vi "VsEP-Compute Final Average.vi"(0 "#Avgs":i32, 1 "Remove DC Offset":bool=TRUE, 5 "Running Sum 1":dbl[](array[numeric]), 9 "Running Sum 2":dbl[](array[numeric]), 11 "AltPol":bool) -> (6 "Neural":dbl[](array[numeric]), 10 "Microphonic":dbl[](array[numeric]))   [LabVIEW 2020]
uses:
  <vilib>/Analysis/baseanly.llb/Mean (DBL).vi
  <vilib>/Analysis/NI_AALBase.lvlib
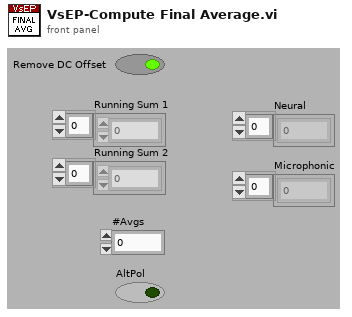
[diagram p1: front panel]
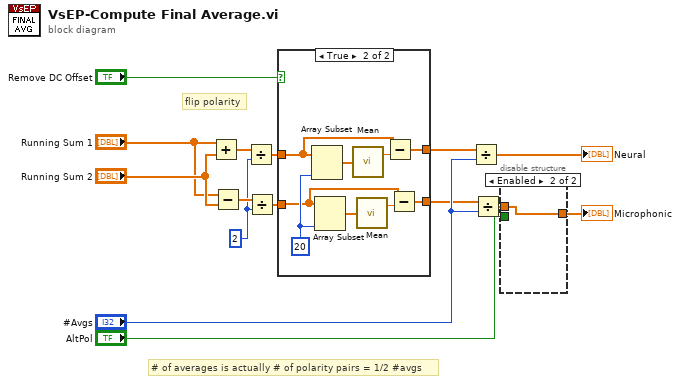
[diagram p0: block diagram]
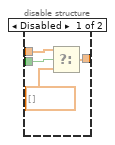
[diagram p3: hidden frame]
diagram:
  w1 = 2
  # "flip polarity"
  # "# of averages is actually # of polarity pairs = 1/2 #avgs"
  n1 = Add(x="Running Sum 1", y="Running Sum 2") -> (x+y=w5:dbl[])
  n2 = Subtract(x="Running Sum 1", y="Running Sum 2") -> (x-y=w4:dbl[])
  n3 = Divide(x=w5, y=w1) -> (x/y=w3:dbl[])
  n4 = Divide(x=w4, y=w1) -> (x/y=w2:dbl[])
  n5 = case shown="True" "Remove DC Offset" {
    tunnel: [w17 w21] -> w8
    tunnel: w3 -> [w17 w22]
    tunnel: [w16 w18] -> w9
    tunnel: w2 -> [w16 w20]
    frame False {
    }
    frame True {
      w26 = 20
      n6 = Array Subset(array=w22, length=w26) -> (w24:dbl[])  [unwired: 1 in]
      n7 = Array Subset(array=w20, length=w26) -> (w25:dbl[])  [unwired: 1 in]
      n8 = call-poly <vilib>:"Mean.vi"("X"=w24) -> ("mean"=w23:dbl)  [unwired: 1 out]
      n9 = call-poly <vilib>:"Mean.vi"("X"=w25) -> ("mean"=w19:dbl)  [unwired: 1 out]
      n10 = Subtract(x=w22, y=w23) -> (x-y=w21:dbl[])
      n11 = Subtract(x=w20, y=w19) -> (x-y=w18:dbl[])
    }
  }
  n12 = Divide(x=w8, y="#Avgs") -> (x/y=→"Neural":dbl[])
  n13 = Divide(x=w9, y="#Avgs") -> (x/y=w11:dbl[])
  n14 = disable-structure shown="Enabled" {
    disable-tunnel: "AltPol" -> [w30 _]
    disable-tunnel: [w28 w31] -> w12
    disable-tunnel: w11 -> [w27 w31]
    frame Disabled {
      n15 = Select(t=w27, s=w30, f=ext[] []) -> (s? t:f=w28:ext[])
    }
    frame Enabled {
    }
  }
  "Microphonic" <- w12
